vi "test Encode and Decoding Parameters for Payload (SGL).vi"() -> ()   [LabVIEW 2020, in "AIM ARINC 664 Scripting.lvclass"]
uses:
  AIM ARINC 664 Scripting.lvclass
  Shared/Encoding (Arinc664).ctl
  <vilib>/addons/_JKI Toolkits/VI Tester/TestCase.llb/TestCase.lvclass
  Engine/Implementation/Rx UDP Execution Unit/Rx UDP Execution Unit.lvclass
  C:/Program Files (x86)/National Instruments/LabVIEW 2020/vi.lib/addons/_JKI Toolkits/VI Tester/TestCase.llb/TestCase.lvclass
panel:
  out "Message Buffer out":u8[](array[numeric])
  out "Data":u8[](array[numeric])
  out "Array":dbl[](array[numeric])
  out "TestCase out":refnum<class "AIM ARINC 664 Scripting.lvclass">
  in  "TestCase in":refnum<class "AIM ARINC 664 Scripting.lvclass">
  out "error out":errorcluster
  in  "error in (no error)":errorcluster
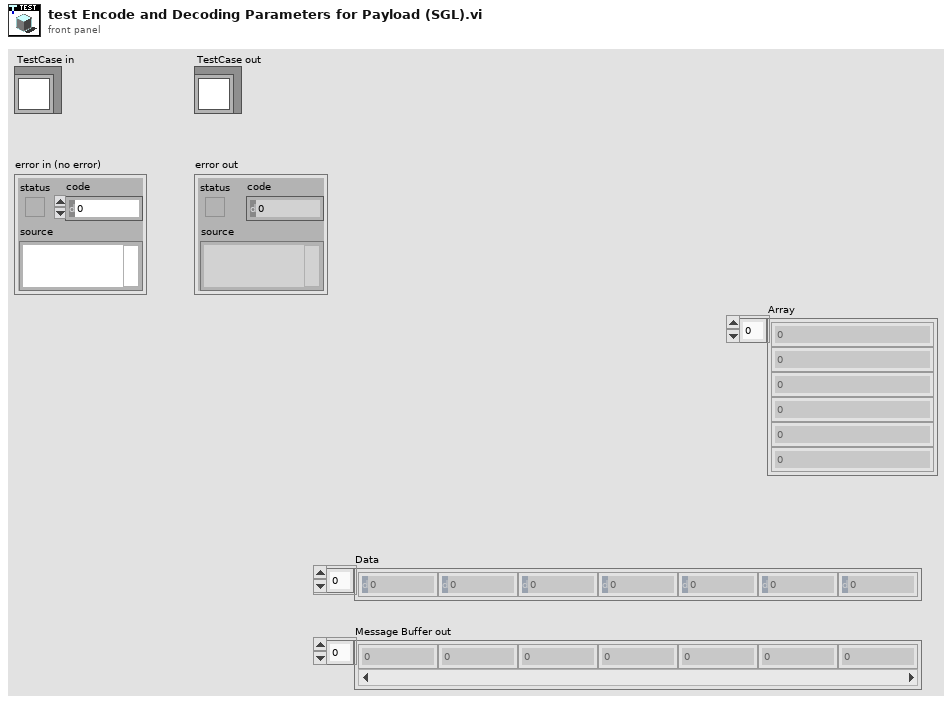
[diagram p1: front panel]
types:
  T1 = typedef "Encoding (Arinc664).ctl" = u16
  T2 = cluster{"start index":i32, "size":i32, "encoding":T1, "signed":bool, "scale multiplier":dbl, "scale offset":dbl}[]
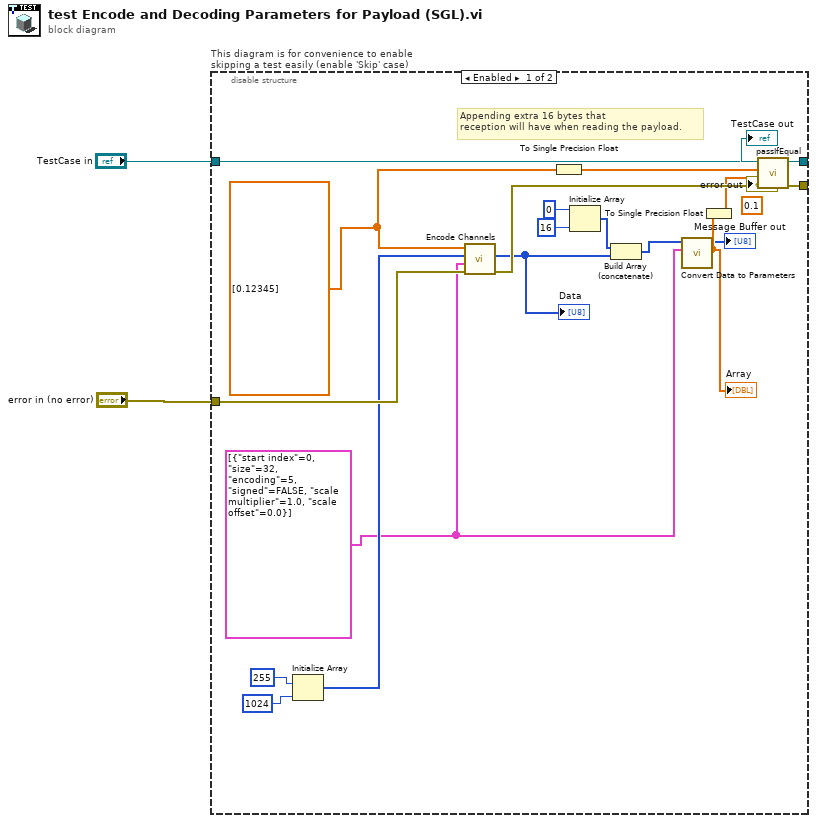
[diagram p0: block diagram]
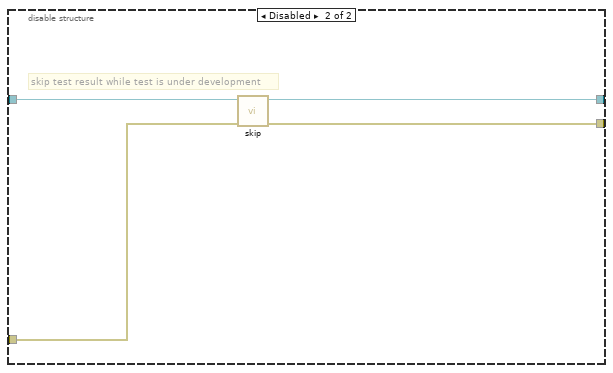
[diagram p2: hidden frame]
diagram:
  n1 = disable-structure "This diagram is for convenience to enable skipping a test easily (enable 'Skip' case)" shown="Enabled" {
    disable-tunnel: "TestCase in" -> [w18 w27]
    disable-tunnel: [w22 w25] -> w2
    disable-tunnel: [w23 w26] -> w3
    disable-tunnel: "error in (no error)" -> [w21 w24]
    frame Enabled {
      w7 = T2 [{"start index"=0, "size"=32, "encoding"=5, "signed"=FALSE, "scale multiplier"=1.0, "scale offset"=0.0}] ("Parameters")
      w8 = dbl[] [0.12345] ("Values in")
      (unwired) 0.1 ("Value")
      # "Appending extra 16 bytes that \nreception will have when reading the payload."
      n2 = Initialize Array(255 ("dimension size"), 1024 ("dimension size")) -> (w9:i32[])
      n3 = call "Encode Channels.vi"("error in"=w21, "Parameters"=w7, "Data in"=w9, "Values in"=w8) -> ("error out"=w17:errorcluster, "Data out"=w10:u8[])  [unwired: 5 in, 1 out]
      "Data" <- w10
      n4 = To Single Precision Float(number=w8) -> (single precision float=w6:sgl[])
      n5 = Initialize Array(0 ("element"), 16 ("dimension size")) -> (w12:i32[])
      n6 = Build Array (concatenate)(w12, w10) -> (w11:i32[])
      n7 = call "Convert Data to Parameters.vi"("Parameters"=w7, "Message Buffer in"=w11) -> ("Array"=w16:dbl[], "Message Buffer out"=→"Message Buffer out":u8[])  [unwired: 8 in]
      "Array" <- w16
      n8 = To Single Precision Float(number=w16) -> (single precision float=w5:sgl[])
      n9 = call-dynamic "passIfEqual.vi"("error in (no error)"=w17, "y"=w5, "x"=w6, "TestCase in"=w18) -> ("error out"=w23:errorcluster, "TestCase out"=w22:refnum<class "AIM ARINC 664 Scripting.lvclass">)  [unwired: 6 in]
    }
    frame Disabled {
      # "skip test result while test is under development"
      n10 = call <vilib>:"skip.vi"("error in (no error)"=w24, "TestCase in"=w27) -> ("error out"=w26:errorcluster, "TestCase out"=w25:refnum<class "AIM ARINC 664 Scripting.lvclass">)  [unwired: 8 in]
    }
  }
  "error out" <- w3
  "TestCase out" <- w2
